vi "Add Execution Monitor Section.vi"(8 "error in":errorcluster, 11 "custom device":T1 format="%.0x") -> (0 "error out":errorcluster, 2 "execution monitor section":T1 format="%.0x", 3 "custom device out":T1 format="%.0x")   [LabVIEW 2020, in "AIM MIL-STD-1553 Scripting.lvlib"]
uses:
  AIM MIL-STD-1553 Scripting.lvlib
  <vilib>/NI VeriStand/Custom Device API/Custom Device Item Ref.ctl
  <vilib>/NI VeriStand/Custom Device API/Custom Device Channel.ctl
  <vilib>/NI VeriStand/Custom Device API/Custom Device Channel Type.ctl
  Constants.vi
  <vilib>/NI VeriStand/Custom Device API/Custom Device API.lvlib
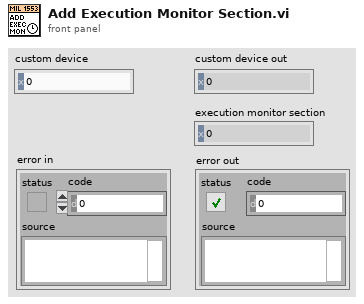
[diagram p1: front panel]
types:
  T1 = typedef "Custom Device API.lvlib/Custom Device Item Ref.ctl" = u64
  T2 = typedef "Custom Device API.lvlib/Custom Device Channel.ctl" = cluster{"Type":T3, "Units":string, "Default Value":dbl, "Faultable":bool, "Scalable":bool}
  T3 = typedef "Custom Device API.lvlib/Custom Device Channel Type.ctl" = enum16{"Input", "Output"}
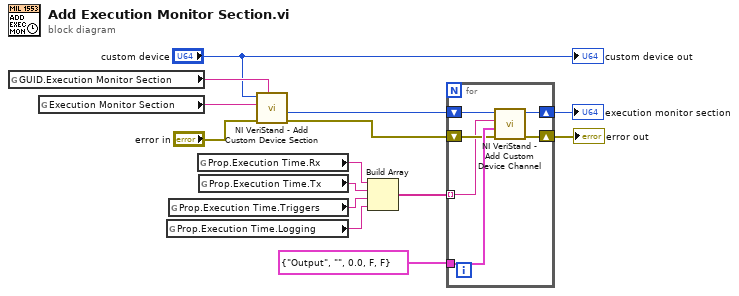
[diagram p0: block diagram]
diagram:
  n1 = global read "Constants.vi" "GUID.Execution Monitor Section"() -> (w14:string)
  n2 = global read "Constants.vi" "Execution Monitor Section"() -> (w13:string)
  n3 = global read "Constants.vi" "Prop.Execution Time.Logging"() -> (w5:string)
  n4 = global read "Constants.vi" "Prop.Execution Time.Triggers"() -> (w4:string)
  n5 = global read "Constants.vi" "Prop.Execution Time.Rx"() -> (w2:string)
  n6 = global read "Constants.vi" "Prop.Execution Time.Tx"() -> (w3:string)
  n7 = call <vilib>:"NI VeriStand - Add Custom Device Section.vi"("GUID (Default Section)"=w14, "error in (no error)"="error in", "Section Name"=w13, "Parent Ref in"="custom device") -> ("error out"=w9:errorcluster, "Section Ptr"=w8:T1)  [unwired: 4 in, 2 out]
  n8 = Build Array(w2, w3, w4, w5) -> (w1:string[])
  n9 = for {
    tunnel: T2 {"Type"=enum."Output", "Units"="", "Default Value"=0.0, "Faultable"=FALSE, "Scalable"=FALSE} ("Channel") -> [w18]
    shift-right: [w19] -> w11
    shift-left: w8 -> [w20]
    shift-right: [w16] -> w6
    shift-left: w9 -> [w17]
    tunnel: w1 -> [w15] mode=indexing
    n10 = call <vilib>:"NI VeriStand - Add Custom Device Channel.vi"("error in (no error)"=w17, "Channel"=w18, "Channel Name"=w15, "Parent Ref in"=w20) -> ("error out"=w16:errorcluster, "Parent Ref out"=w19:T1)  [unwired: 4 in, 2 out]
  }
  "execution monitor section" <- w11
  "error out" <- w6
  "custom device out" <- "custom device"
